vi "Plug_in_data_global.vi"() -> ()   [LabVIEW 2020]
panel:
  in  "Plug_in Folder depth":i32
  in  "Plug_in Results Folder":path
  out "Templated Results header":string[][](array[string])
  out "Results File Plotter Rows":string[][](array[string])
  in  "FFID Bkgnd Values":dbl[](array[numeric])
  in  "Block Header":string
  in  "Server Channels to log":string[](array[string])
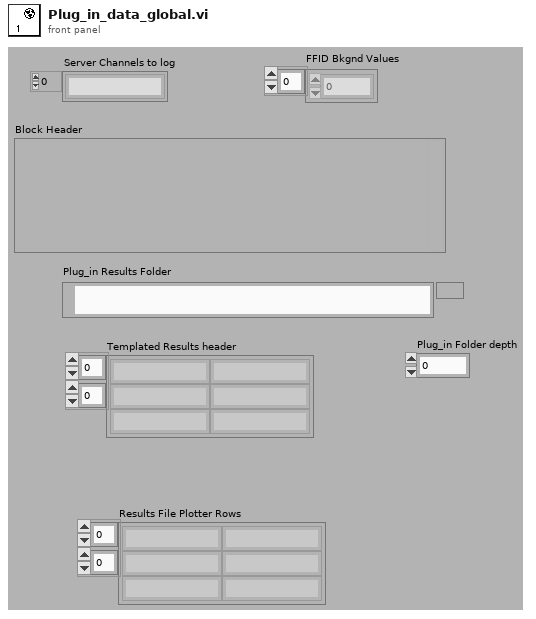
[diagram p1: front panel]
diagram:
